vi "setupILC.vi"(8 "error in (no error)":errorcluster, 10 "Model in":refnum<class "Model.lvclass">, 11 "Bootloader in":refnum<class "Bootloader.lvclass">) -> (0 "error out":errorcluster, 2 "Model out":refnum<class "Model.lvclass">, 3 "Bootloader out":refnum<class "Bootloader.lvclass">)   [LabVIEW 2015, in "Bootloader.lvclass"]
uses:
  Bootloader.lvclass
  Model/Model.lvclass
  <userlib>/Common/SerialProtocols/SerialProtocolFactory/SerialProtocolFactory/SerialProtocolFactory.lvclass
  <userlib>/Common/SerialProtocols/SerialCommunicator/SerialCommunicator.lvclass
  ILCTC/ILCTC.lvclass
  <userlib>/Common/SerialProtocols/SerialCommunicator/SerialCommunicator.lvclass/SerialCommunicator.ctl
  <userlib>/Common/ILC/ILC/ILC.lvclass/ILC.ctl
  Model/Model.lvclass/Model.ctl
  <userlib>/Common/ILC/ILC/ILC.lvclass
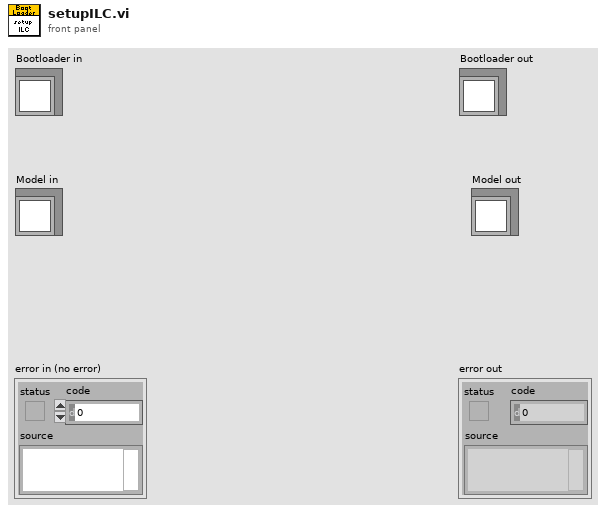
[diagram p1: front panel]
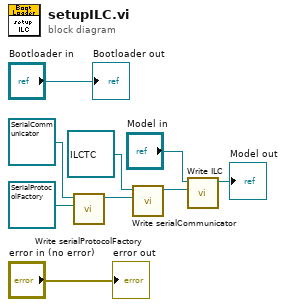
[diagram p0: block diagram]
diagram:
  n1 = call <userlib>:"Write serialProtocolFactory.vi"("serialProtocolFactory"=refnum<class "SerialProtocolFactory.lvclass"> refnum ("SerialCommFactory.lvclass"), "SerialCommunicator in"=refnum<class "SerialCommunicator.lvclass"> refnum ("SerialProtocols.lvlib:SerialCommunicator.lvclass")) -> ("SerialCommunicator out"=w5:refnum<class "SerialCommunicator.lvclass">)  [unwired: 9 in]
  n2 = call <userlib>:"Write serialCommunicator.vi"("serialCommunicator"=w5, "ILC in"=refnum<class "ILCTC.lvclass"> refnum ("ILC_TC.lvclass")) -> ("ILC out"=w3:refnum<class "ILCTC.lvclass">)  [unwired: 9 in]
  n3 = call "Write ILC.vi"("ilc"=w3, "Model in"="Model in") -> ("Model out"=→"Model out":refnum<class "Model.lvclass">)  [unwired: 9 in]
  "error out" <- "error in (no error)"
  "Bootloader out" <- "Bootloader in"
